vi "ZS_DPLab_Main_ver3.1.vi"() -> ()   [LabVIEW 2011]
panel:
  in  "File type":u16(ring) items=["Txt"=0, "Both"=2]
  out "StartTime(ms)":u32
  in  "Pause":bool
  in  "stop":bool
  in  "Main Sweep":u8(ring) items=["Time", "DC Current", "Delta Current", "Pulse Delta Current", "Sine Current", "Lock-In Vosc"]
  out "Run index":string
  in  "File Index:":u16=1 format="%03d"
  out "TakingData":bool
  in  "Data File Address":path
  in  "Tab Control":T1(tab)
  in  "Steps Config:":T2={"# of points:"=100, "Step Delay (s)"=1.0, "Ini Delay (s)"=3.0, "# of steps:"=1} {"# of steps:" step=1; "# of points:" step=1; "Step Delay (s)" min=0.0 format="%3.2f"; "Ini Delay (s)" min=0.0 format="%3.2f"}
  in  "Tab Control 2":enum32{"ITC 503", "LS 340"}(tab)
  in  "Temperature Control (ITC 503):":T3={"GPIB ADR"=0, "Change Heater?"={"Change Heater?"=FALSE, "Heater"=0}, "Change Temp?"={"Change Temp?"=FALSE, "Set Temp (K)"=0.0}, "Cluster"={"Heat Auto?"=FALSE, "Manual Heat?"=FALSE, "Heater Manual (%)"=0.0}, "Change PID?"={"Change PID?"=FALSE, "Proportional"=0.0, "Integral"=0.0, "Derivative"=0.0}, "Change Para?"=FALSE, "ITC503 Control Sensor"=1} {"ITC503 Control Sensor" items=["T2", "T3"]; "Change PID?"."Derivative" format="%.2f"; "Change PID?"."Integral" format="%.2f"; "Change PID?"."Proportional" format="%.2f"; "Cluster"."Heater Manual (%)" scale=0.0..100.0; "Change Temp?"."Set Temp (K)" format="%.3f"; "Change Heater?"."Heater" items=["Heater 1", "Heater 2", "Heater 3"]; "GPIB ADR" items=["None"=0, "24"=24]}
  in  "Temperature Control (LS 340):":T4={"GPIB ADR"=0, "From (K)"=0.0, "To (K)"=0.0, "Rate (K/min; 0~100)"=1.0, "Delta T (0.08K)"=0.08, "Temp. Header"="Temp_K", "Temp. Display controller"={"Ch B"=TRUE, "Ch C"=TRUE, "Ch D"=FALSE}} {"Delta T (0.08K)" format="%.3f"; "Rate (K/min; 0~100)" format="%.1f"; "To (K)" format="%.2f"; "From (K)" format="%.2f"; "GPIB ADR" items=["None"=0, "30"=30]}
  in  "Measuring Instruments :":T5(array[cluster])
  in  "Keithley 6221 :":T6(array[cluster]) {"Sweep Mode" items=["Linear", "Log", "Exp", "Inverse", "Manual"]; "GPIB ADR" items=["None"=0, "12"=12, "13"=13]; "To I_Sin (A)" format="%#.5p"; "To I_H (A)" format="%#.5p"; "To I_HI (A)" format="%#.5p"; "To I (A)" format="%#.5p"; "Delay (s)" format="%.3p"; "Pulse Width (s)" format="%.3p"; "Delay Time (s)" format="%#.5p"; "DC Offset (A)" format="%#.5p"; "From I_Sin (A)" format="%#.5p"; "Freq (Hz)" format="%#_6p"; "I_L (A)" format="%#.5p"; "From I_H (A)" format="%#.5p"; "I_LO (A)" format="%#.5p"; "From I (A)" format="%#.5p"; "From I_HI (A)" format="%#.5p"}
  in  "Lock-In SR7265 :":T7(array[cluster]) {"Sweep Mode" items=["Linear", "Log", "Exp", "Inverse", "Manual"]; "To" format="%#.5p"; "From" format="%#.5p"; "GPIB ADR" items=["None"=0, "11"=11, "16"=16]}
  in  "Description of this measurement":string
  in  "Varialbe Instruments:":i32(listbox)
  in  "Instruments Config:":string[][](table) caption="Table"
  out "Configuration Profile:":string
  in  "Up Button":bool
  in  "Delete Button":bool
  in  "Down Button":bool
  in  "Add one Run":bool
  in  "Tab Control 3":enum32{"ReadMe", "Control Panel"}(tab)
  in  "Magnet Control (IPS 120-10)":T8={"Action"=1, "Standby (s)"=0.0, "Heater on (s)"=300.0, "Sweep Setup "=[], "GPIB ADR"=0, "Change Para?"=FALSE} {"GPIB ADR" items=["None"=0, "25"=25]; "Sweep Setup"."Hold(min)" min=0.0; "Sweep Setup"."Set Rate(T/min)" min=0.001 max=0.5 step=0.001; "Sweep Setup"."Set Point (T)" min=-9.0 max=9.0 step=0.001; "Action" items=["Hold", "To Set Point", "To Zero", "Clamp"]}
  in  "SettingGo":bool
  in  "Discarded pts":i32
  in  "Analysis":bool=TRUE
  in  "Measure with H/T sweep?":bool=TRUE
  in  "Run Batch Array":T9(array[cluster]) {"Main Sweep" items=["Time", "DC Current", "Delta Current", "Pulse Delta Current", "Sine Current", "Lock-in Vosc"]; "Temperature Control (ITC 503):"."Sensor" items=["T2", "T3"]; "Magnet Control (IPS 120-10)"."Action" items=["Hold", "To Set point", "To Zero", "Clamp"]; "Keithley 6221 :"."Sweep Mode" items=["Linear", "Log", "Exp", "Inverse", "Manual"]}
  in  "Delete Run":bool
  in  "BatchSettingGo":bool
  out "T2":string
  out "T3":string
  out "B":string
  out "T1":string
  in  "DisplayControl":T10 {"Scale" items=["L", "R"]; "Y - axes"."Y 6" items=["", "Time_sec", "T2_K", "T3_K", "I_DeltaHigh_A", "V_Delta_V", "CernoxV_V"]; "Y - axes"."Y 5" items=["", "Time_sec", "T2_K", "T3_K", "I_DeltaHigh_A", "V_Delta_V", "CernoxV_V"]; "Y - axes"."Y 4" items=["", "Time_sec", "T2_K", "T3_K", "I_DeltaHigh_A", "V_Delta_V", "CernoxV_V"]; "Y - axes"."Y 3" items=["", "Time_sec", "T2_K", "T3_K", "I_DeltaHigh_A", "V_Delta_V", "CernoxV_V"]; "Y - axes"."Y 2" items=["", "Time_sec", "T2_K", "T3_K", "I_DeltaHigh_A", "V_Delta_V", "CernoxV_V"]; "Y - axes"."Y 1" items=["", "Time_sec", "T2_K", "T3_K", "I_DeltaHigh_A", "V_Delta_V", "CernoxV_V"]; "X - axis" items=["Time_sec", "T2_K", "T3_K", "I_DeltaHigh_A", "V_Delta_V", "CernoxV_V"]}
  out "XY Graph":cluster{"DataOut":dbl[], "DataOut":dbl[]}[](graph)
  out "DataDisplay":T11
  out "Set T:":string
  out "Set B:":string
  out "Title Name Array":string[](array[string])
  out "Data Table":dbl[][](array[numeric])
  out "XY Graph 2":cluster{"DataOut":dbl[], "DataOut":dbl[]}[](graph)
  in  "AnalysisDisplayControl":T10 {"Scale" items=["L", "R"]; "Y - axes"."Y 6" items=["", "Time_sec", "T2_K", "Std_T2_K", "T3_K", "Std_T3_K", "I_DeltaHigh_A", "Std_I_DeltaHigh_A", "V_Delta_V", "Std_V_Delta_V", "CernoxV_V", "Std_CernoxV_V", "CernoxR_Ohms", "Std_CernoxR_Ohms", "CernoxT_K", "Std_CernoxT_K"]; "Y - axes"."Y 5" items=["", "Time_sec", "T2_K", "Std_T2_K", "T3_K", "Std_T3_K", "I_DeltaHigh_A", "Std_I_DeltaHigh_A", "V_Delta_V", "Std_V_Delta_V", "CernoxV_V", "Std_CernoxV_V", "CernoxR_Ohms", "Std_CernoxR_Ohms", "CernoxT_K", "Std_CernoxT_K"]; "Y - axes"."Y 4" items=["", "Time_sec", "T2_K", "Std_T2_K", "T3_K", "Std_T3_K", "I_DeltaHigh_A", "Std_I_DeltaHigh_A", "V_Delta_V", "Std_V_Delta_V", "CernoxV_V", "Std_CernoxV_V", "CernoxR_Ohms", "Std_CernoxR_Ohms", "CernoxT_K", "Std_CernoxT_K"]; "Y - axes"."Y 3" items=["", "Time_sec", "T2_K", "Std_T2_K", "T3_K", "Std_T3_K", "I_DeltaHigh_A", "Std_I_DeltaHigh_A", "V_Delta_V", "Std_V_Delta_V", "CernoxV_V", "Std_CernoxV_V", "CernoxR_Ohms", "Std_CernoxR_Ohms", "CernoxT_K", "Std_CernoxT_K"]; "Y - axes"."Y 2" items=["", "Time_sec", "T2_K", "Std_T2_K", "T3_K", "Std_T3_K", "I_DeltaHigh_A", "Std_I_DeltaHigh_A", "V_Delta_V", "Std_V_Delta_V", "CernoxV_V", "Std_CernoxV_V", "CernoxR_Ohms", "Std_CernoxR_Ohms", "CernoxT_K", "Std_CernoxT_K"]; "Y - axes"."Y 1" items=["", "Time_sec", "T2_K", "Std_T2_K", "T3_K", "Std_T3_K", "I_DeltaHigh_A", "Std_I_DeltaHigh_A", "V_Delta_V", "Std_V_Delta_V", "CernoxV_V", "Std_CernoxV_V", "CernoxR_Ohms", "Std_CernoxR_Ohms", "CernoxT_K", "Std_CernoxT_K"]; "X - axis" items=["Time_sec", "T2_K", "Std_T2_K", "T3_K", "Std_T3_K", "I_DeltaHigh_A", "Std_I_DeltaHigh_A", "V_Delta_V", "Std_V_Delta_V", "CernoxV_V", "Std_CernoxV_V", "CernoxR_Ohms", "Std_CernoxR_Ohms", "CernoxT_K", "Std_CernoxT_K"]}
  in  "Cernox T Fitting Control":T12={"Cernox V title"="CernoxV_V", "Cernox I title"="CernoxI_V", "Cernox V Lockin Sen (V)"=0.001, "Cernox I Lockin Sensitivity (V)"=0.02, "Cernox I Current Amp Sen (A/V)"=1e-05, "Cernox Fit"=TRUE}
  in  "CernoxI measured with a lock-in?":bool
  in  "Cernox_I":dbl=4.965
  # "If set rate = 0,                           Ramping is off."
  # "If set temp. = 0,    \nThe Temp. is not controlled."
  # "Before you start:\n1. Make sure you finished the training and authorized to use this magnet.\n2. Check Helium level of the cryostat before you proceed. Generally you should sweep field back to zero if the level is below 16%.\n3. This module is designed for normal sweep mode, so make sure the \"SWITCH HEATER\" is \"SELECT\" and \"CONFIRM\". If you need the persistent mode, please control IPS manualy.\n4. This module is adopted from Xiaoyan_IPS_120_10 ver2.0-2.vi. Please make sure you are absolutely familiar with all the settings before you start to set up the batch files.\n5. Recommended B sweep rate is ~ 0.1 T/min."
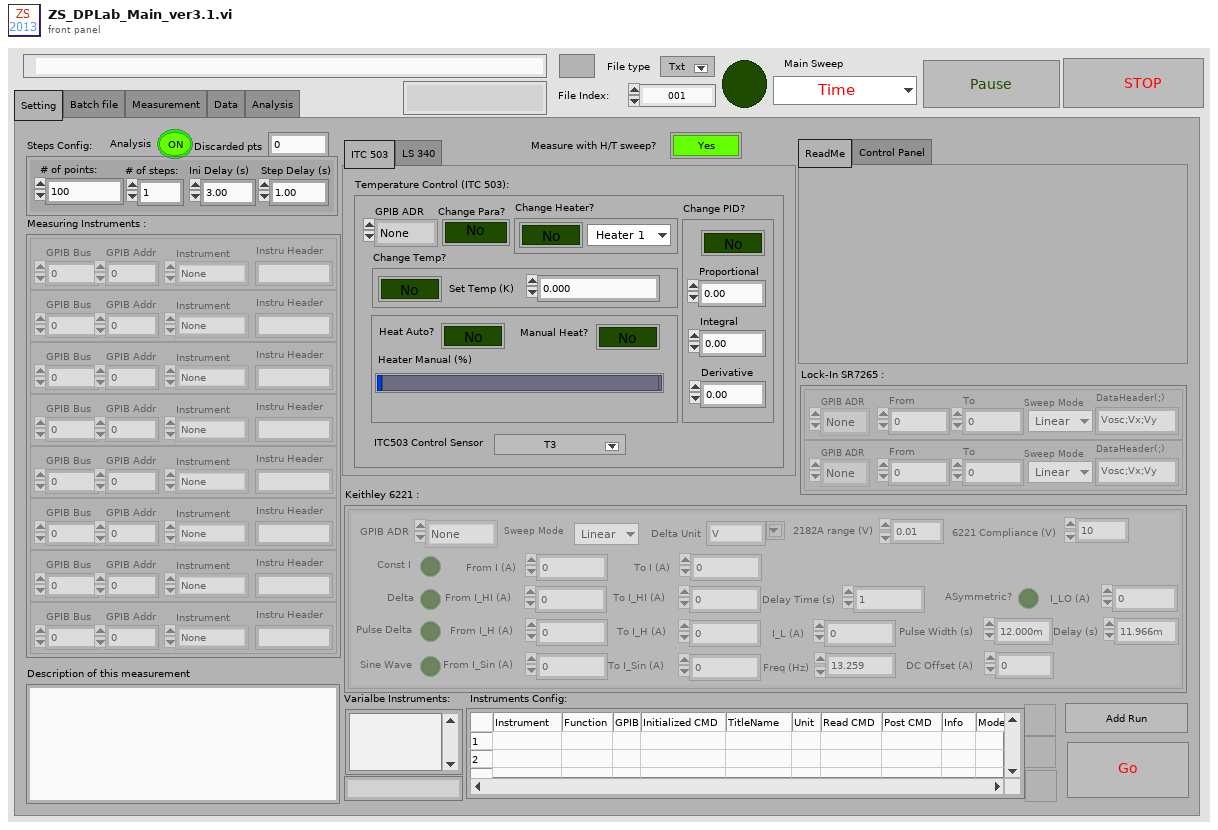
[diagram p1: front panel]
types:
  T1 = enum32{"Setting", "Batch file", "Measurement", "Data", "Analysis"}
  T2 = cluster{"# of points:":u32, "Step Delay (s)":dbl, "Ini Delay (s)":dbl, "# of steps:":u32}
  T3 = cluster{"GPIB ADR":u16, "Change Heater?":cluster{"Change Heater?":bool, "Heater":u8}, "Change Temp?":cluster{"Change Temp?":bool, "Set Temp (K)":dbl}, "Cluster":cluster{"Heat Auto?":bool, "Manual Heat?":bool, "Heater Manual (%)":dbl}, "Change PID?":cluster{"Change PID?":bool, "Proportional":dbl, "Integral":dbl, "Derivative":dbl}, "Change Para?":bool, "ITC503 Control Sensor":u16}
  T4 = cluster{"GPIB ADR":u16, "From (K)":dbl, "To (K)":dbl, "Rate (K/min; 0~100)":dbl, "Delta T (0.08K)":dbl, "Temp. Header":string, "Temp. Display controller":cluster{"Ch B":bool, "Ch C":bool, "Ch D":bool}}
  T5 = cluster{"GPIB Bus":dbl, "GPIB Addr":dbl, "Instrument":enum16{"None", "HP34401DMM", "Lockin 7265", "HP3456/7A", "HP3478A", "HP3325FG", "Keithley2182A"}, "Instru Header":string}[]
  T6 = cluster{"Delta ":bool, "Const I ":bool, "Pulse Delta ":bool, "Sine Wave ":bool, "From I_HI (A)":dbl, "From I (A)":dbl, "I_LO (A)":dbl, "From I_H (A)":dbl, "I_L (A)":dbl, "Freq (Hz)":dbl, "From I_Sin (A)":dbl, "DC Offset (A)":dbl, "Delay Time (s)":dbl, "Pulse Width (s)":dbl, "Delay (s)":dbl, "To I (A)":dbl, "ASymmetric?":bool, "To I_HI (A)":dbl, "To I_H (A)":dbl, "To I_Sin (A)":dbl, "GPIB ADR":u16, "Sweep Mode":u8, "Delta Unit":string, "2182A range (V)":dbl, "6221 Compliance (V)":dbl}[]
  T7 = cluster{"GPIB ADR":u16, "From":dbl, "To":dbl, "DataHeader(;)":string, "Sweep Mode":u8}[]
  T8 = cluster{"Action":u16, "Standby (s)":dbl, "Heater on (s)":dbl, "Sweep Setup ":cluster{"Set Point (T)":dbl, "Set Rate(T/min)":dbl, "Hold(min)":dbl}[], "GPIB ADR":u16, "Change Para?":bool}
  T9 = cluster{"Main Sweep":u8, "Steps Config:":cluster{"total points:":u32, "Step Delay (s)":dbl, "Ini Delay (s)":dbl, "# of steps:":u32}, "Temperature Control (ITC 503):":cluster{"GPIB ADR":u16, "Change Heater?":cluster{"Heater?":bool, "Heater":u8}, "Change Temp?":cluster{"Change T?":bool, "Set T (K)":dbl}, "Cluster":cluster{"Heat Auto?":bool, "Manual Heat?":bool, "Heater (%)":dbl}, "Change PID?":cluster{"Change PID?":bool, "P":dbl, "I":dbl, "D":dbl}, "Change Para?":bool, "Sensor":u16}, "Temperature Control (LS 340):":cluster{"GPIB ADR":u16, "From (K)":dbl, "To (K)":dbl, "Rate (K/min)":dbl, "Delta T (0.08K)":dbl, "Temp. Header":string, "T Display Control":cluster{"Ch B":bool, "Ch C":bool, "Ch D":bool}}, "Magnet Control (IPS 120-10)":cluster{"Action":u16, "Standby (s)":dbl, "Heater on (s)":dbl, "Sweep Setup ":cluster{"Set Point (T)":dbl, "Set Rate(T/min)":dbl, "Hold(min)":dbl}[], "GPIB ADR":u16, "Change Para?":bool}, "Keithley 6221 :":cluster{"Delta mode":bool, "Const I":bool, "Pulse Delta mode":bool, "Sine Wave Mode":bool, "From I_HI (A)":dbl, "From I (A)":dbl, "I_LO (A)":dbl, "From I_H (A)":dbl, "I_L (A)":dbl, "Freq (Hz)":dbl, "From I_Sin (A)":dbl, "DC Offset (A)":dbl, "Delay Time (s)":dbl, "Pulse Width (s)":dbl, "Delay (s)":dbl, "To I (A)":dbl, "ASymmetric?":bool, "To I_HI (A)":dbl, "To I_H (A)":dbl, "To I_Sin (A)":dbl, "GPIB ADR":u16, "Sweep Mode":u8, "Delta Unit":string, "2182A range (V)":dbl, "6221 Compliance (V)":dbl}[], "Measuring Instruments : ":cluster{"GPIB Bus":dbl, "GPIB Addr":dbl, "Instrument":enum16{"None", "HP34401DMM", "Lockin 7265", "HP3456/7A", "HP3478A", "HP3325FG", "Keithley2182A"}, "Instru Header":string}[], "Lock-In SR7265 :":cluster{"GPIB ADR":u16, "From":dbl, "To":dbl, "Header(;)":string, "Sweep Mode":u8}[], "Deascription of \nthis measurement":string, "Instruments Config:":string[][]}[]
  T10 = cluster{"X - axis":u8, "Y - axes":cluster{"Y 1":u8, "Y 2":u8, "Y 3":u8, "Y 4":u8, "Y 5":u8, "Y 6":u8}, "Scale":u16[]}
  T11 = cluster{"X":dbl, "Y 1":dbl, "Y 2":dbl, "Y 3":dbl, "Y 4":dbl, "Y 5":dbl, "Y 6":dbl}
  T12 = cluster{"Cernox V title":string, "Cernox I title":string, "Cernox V Lockin Sen (V)":dbl, "Cernox I Lockin Sensitivity (V)":dbl, "Cernox I Current Amp Sen (A/V)":dbl, "Cernox Fit":bool}
  T13 = cluster{"Main Sweep":u8, "Steps Config:":cluster{"total points:":u32, "Step Delay (s)":dbl, "Ini Delay (s)":dbl, "# of steps:":u32}, "Temperature Control (ITC 503):":cluster{"GPIB ADR":u16, "Change Heater?":cluster{"Heater?":bool, "Heater":u8}, "Change Temp?":cluster{"Change T?":bool, "Set T (K)":dbl}, "Cluster":cluster{"Heat Auto?":bool, "Manual Heat?":bool, "Heater (%)":dbl}, "Change PID?":cluster{"Change PID?":bool, "P":dbl, "I":dbl, "D":dbl}, "Change Para?":bool, "Sensor":u16}, "Temperature Control (LS 340):":cluster{"GPIB ADR":u16, "From (K)":dbl, "To (K)":dbl, "Rate (K/min)":dbl, "Delta T (0.08K)":dbl, "Temp. Header":string, "T Display Control":cluster{"Ch B":bool, "Ch C":bool, "Ch D":bool}}, "Magnet Control (IPS 120-10)":cluster{"Action":u16, "Standby (s)":dbl, "Heater on (s)":dbl, "Sweep Setup ":cluster{"Set Point (T)":dbl, "Set Rate(T/min)":dbl, "Hold(min)":dbl}[], "GPIB ADR":u16, "Change Para?":bool}, "Keithley 6221 :":cluster{"Delta mode":bool, "Const I":bool, "Pulse Delta mode":bool, "Sine Wave Mode":bool, "From I_HI (A)":dbl, "From I (A)":dbl, "I_LO (A)":dbl, "From I_H (A)":dbl, "I_L (A)":dbl, "Freq (Hz)":dbl, "From I_Sin (A)":dbl, "DC Offset (A)":dbl, "Delay Time (s)":dbl, "Pulse Width (s)":dbl, "Delay (s)":dbl, "To I (A)":dbl, "ASymmetric?":bool, "To I_HI (A)":dbl, "To I_H (A)":dbl, "To I_Sin (A)":dbl, "GPIB ADR":u16, "Sweep Mode":u8, "Delta Unit":string, "2182A range (V)":dbl, "6221 Compliance (V)":dbl}[], "Measuring Instruments : ":cluster{"GPIB Bus":dbl, "GPIB Addr":dbl, "Instrument":enum16{"None", "HP34401DMM", "Lockin 7265", "HP3456/7A", "HP3478A", "HP3325FG", "Keithley2182A"}, "Instru Header":string}[], "Lock-In SR7265 :":cluster{"GPIB ADR":u16, "From":dbl, "To":dbl, "Header(;)":string, "Sweep Mode":u8}[], "Deascription of \nthis measurement":string, "Instruments Config:":string[][]}
  T14 = enum32{"Setting", "Batch file", "Measurement", "Data"}
  T15 = cluster{"Main Sweep":u8, "Steps Config:":cluster{"# of points:":u32, "Step Delay (s)":dbl, "Ini Delay (s)":dbl, "# of steps:":u32}, "Temperature Control (ITC 503):":cluster{"GPIB ADR":u16, "Change Heater?":cluster{"Change Heater?":bool, "Heater":u8}, "Change Temp?":cluster{"Change Temp?":bool, "Set Temp (K)":dbl}, "Cluster":cluster{"Heat Auto?":bool, "Manual Heat?":bool, "Heater Manual (%)":dbl}, "Change PID?":cluster{"Change PID?":bool, "Proportional":dbl, "Integral":dbl, "Derivative":dbl}, "Change Para?":bool, "ITC503 Control Sensor":u16}, "Temperature Control (LS 340):":cluster{"GPIB ADR":u16, "From (K)":dbl, "To (K)":dbl, "Rate (K/min; 0~100)":dbl, "Delta T (0.08K)":dbl, "Temp. Header":string, "Temp. Display controller":cluster{"Ch B":bool, "Ch C":bool, "Ch D":bool}}, "Magnet Control (IPS 120-10)":cluster{"Action":u16, "Standby (s)":dbl, "Heater on (s)":dbl, "Sweep Setup ":cluster{"Set Point (T)":dbl, "Set Rate(T/min)":dbl, "Hold(min)":dbl}[], "GPIB ADR":u16, "Change Para?":bool}, "Keithley 6221 :":cluster{"Delta ":bool, "Const I ":bool, "Pulse Delta ":bool, "Sine Wave ":bool, "From I_HI (A)":dbl, "From I (A)":dbl, "I_LO (A)":dbl, "From I_H (A)":dbl, "I_L (A)":dbl, "Freq (Hz)":dbl, "From I_Sin (A)":dbl, "DC Offset (A)":dbl, "Delay Time (s)":dbl, "Pulse Width (s)":dbl, "Delay (s)":dbl, "To I (A)":dbl, "ASymmetric?":bool, "To I_HI (A)":dbl, "To I_H (A)":dbl, "To I_Sin (A)":dbl, "GPIB ADR":u16, "Sweep Mode":u8, "Delta Unit":string, "2182A range (V)":dbl, "6221 Compliance (V)":dbl}[], "Measuring Instruments : ":cluster{"GPIB Bus":dbl, "GPIB Addr":dbl, "Instrument":enum16{"None", "HP34401DMM", "Lockin 7265", "HP3456/7A", "HP3478A", "HP3325FG", "Keithley2182A"}, "Instru Header":string}[], "Lock-In SR7265 :":cluster{"GPIB ADR":u16, "From":dbl, "To":dbl, "DataHeader(;)":string, "Sweep Mode":u8}[], "Description of this measurement":string, "Instruments Config:":string[][]}
  T16 = typedef "LVRowAndColumnTypeDef.ctl" = cluster{"Row":i32, "Column":i32}
  T17 = cluster{"Delta mode":bool, "Const I":bool, "Pulse Delta mode":bool, "Sine Wave Mode":bool, "From I_HI (A)":dbl, "From I (A)":dbl, "I_LO (A)":dbl, "From I_H (A)":dbl, "I_L (A)":dbl, "Freq (Hz)":dbl, "From I_Sin (A)":dbl, "DC Offset (A)":dbl, "Delay Time (s)":dbl, "Pulse Width (s)":dbl, "Delay (s)":dbl, "To I (A)":dbl, "ASymmetric?":bool, "To I_HI (A)":dbl, "To I_H (A)":dbl, "To I_Sin (A)":dbl, "GPIB ADR":u16, "Sweep Mode":u8, "Delta Unit":string, "2182A range (V)":dbl, "6221 Compliance (V)":dbl}[]
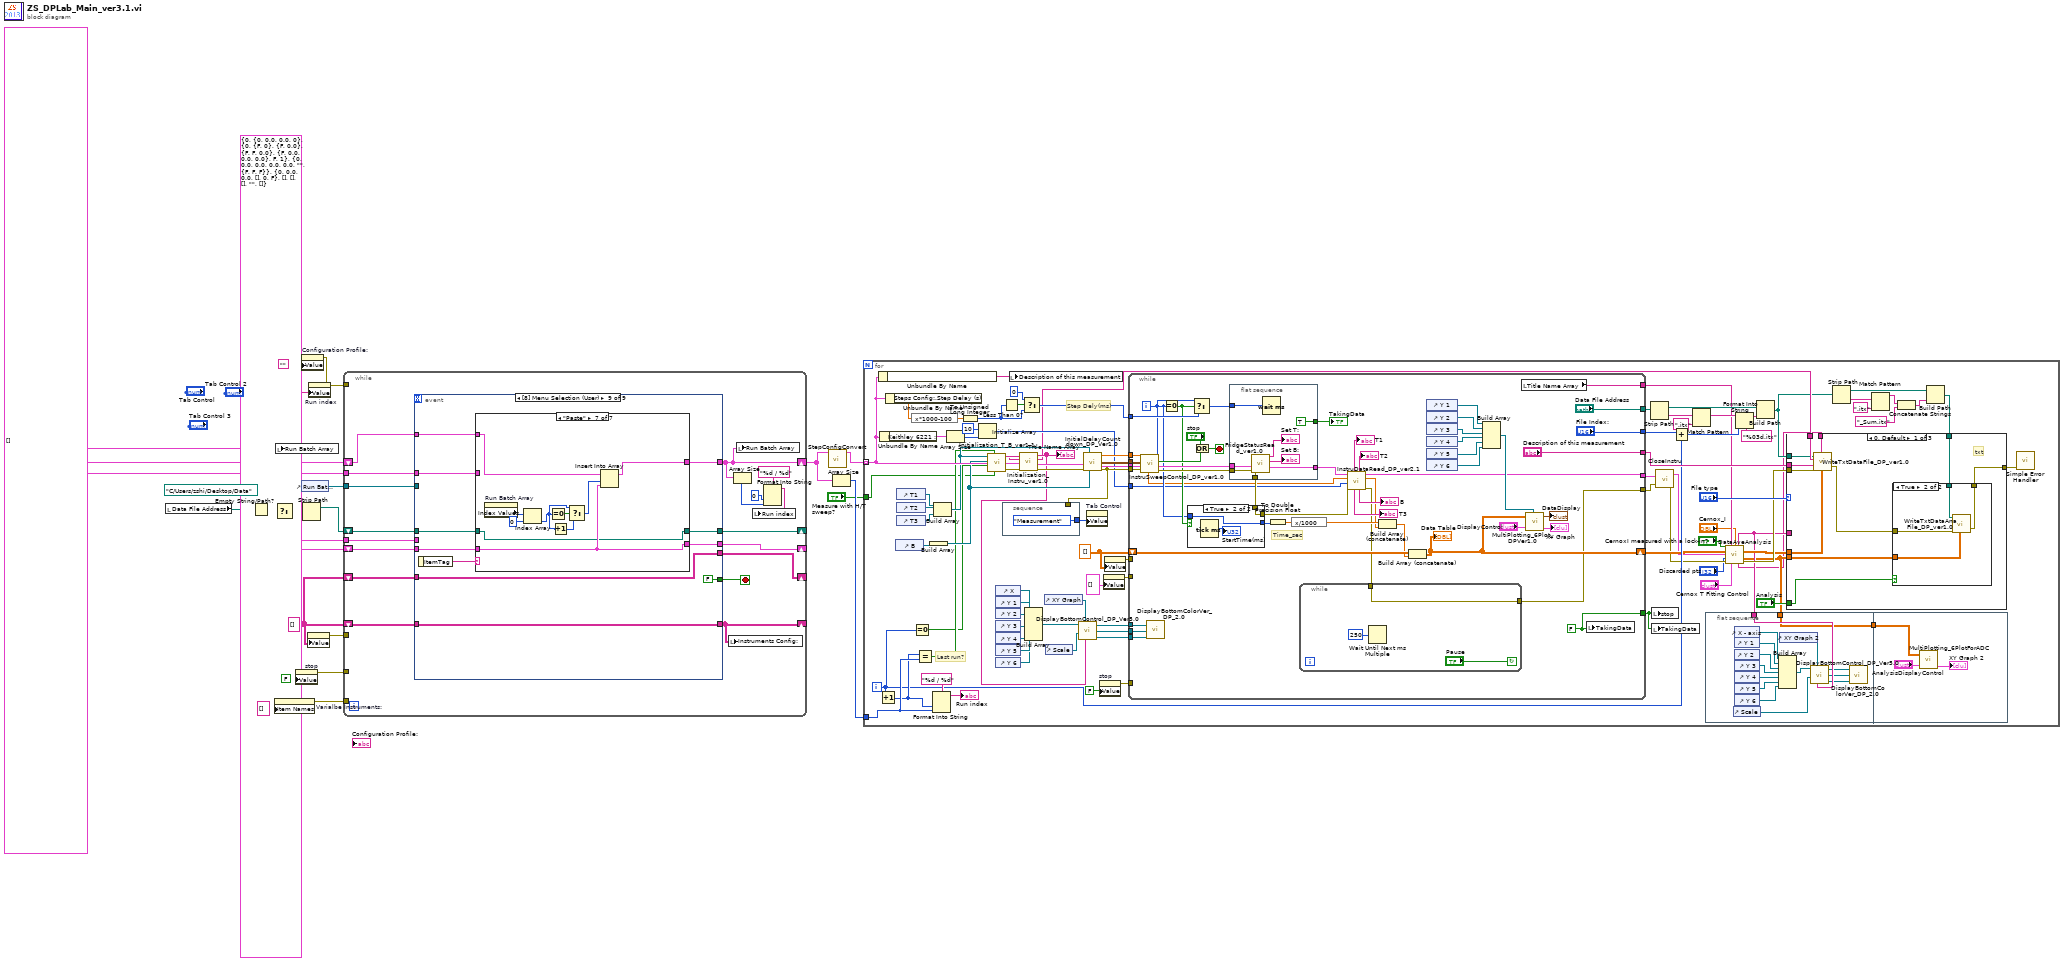
[diagram p0: block diagram]
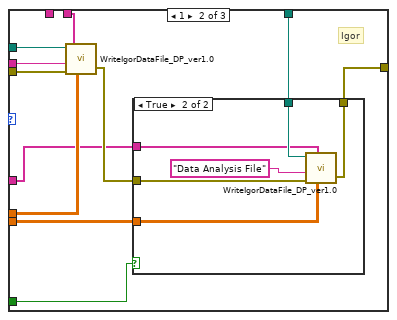
[diagram p3: hidden frame]
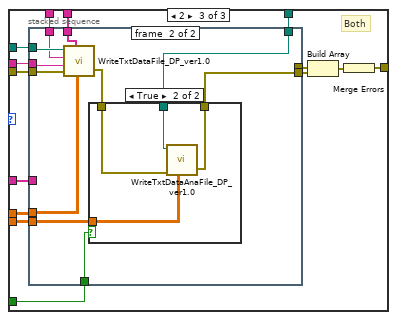
[diagram p5: hidden frame]
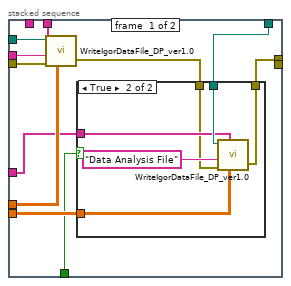
[diagram p6: hidden frame]
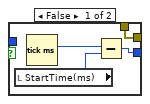
[diagram p9: hidden frame]
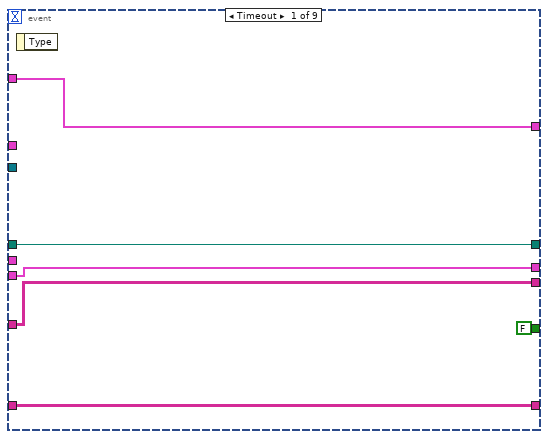
[diagram p10: hidden frame]
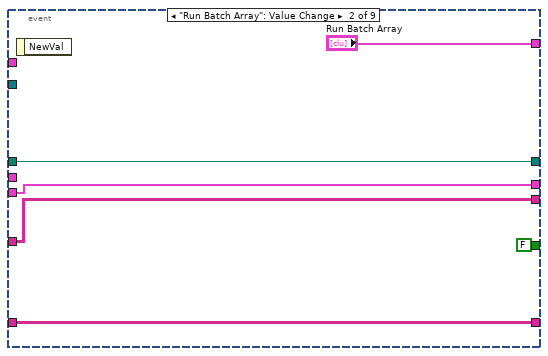
[diagram p11: hidden frame]
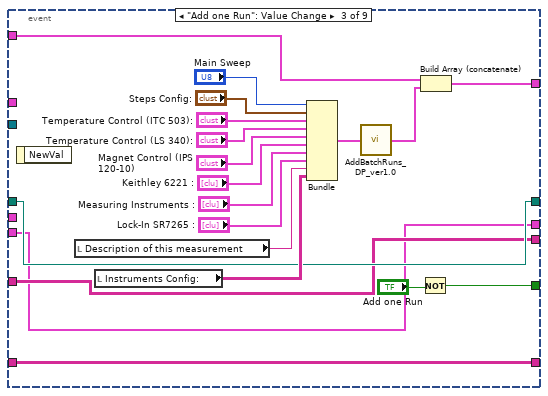
[diagram p12: hidden frame]
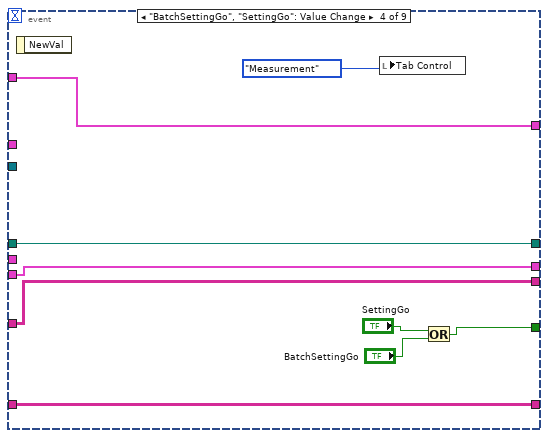
[diagram p13: hidden frame]
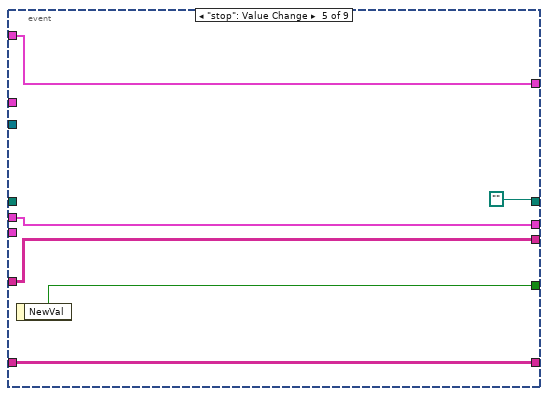
[diagram p14: hidden frame]
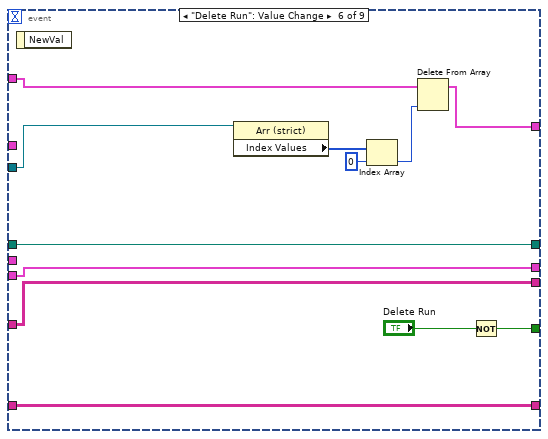
[diagram p15: hidden frame]
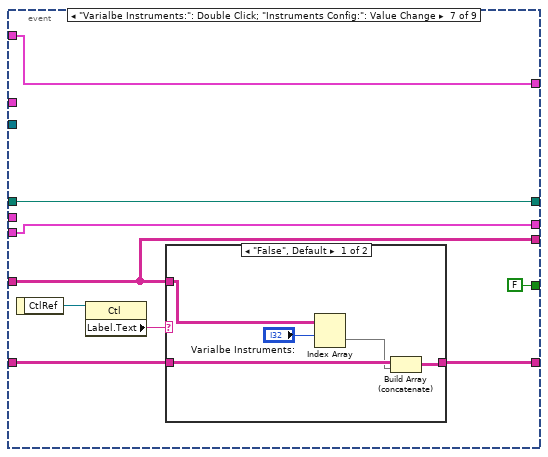
[diagram p16: hidden frame]
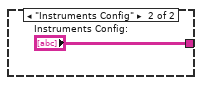
[diagram p17: hidden frame]
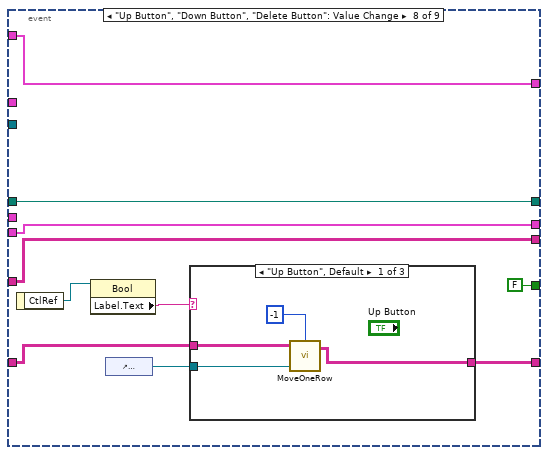
[diagram p18: hidden frame]
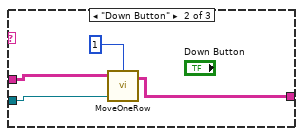
[diagram p19: hidden frame]
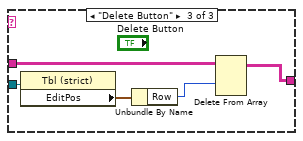
[diagram p20: hidden frame]
diagram:
  w2 = T13 {"Main Sweep"=0, "Steps Config:"={"total points:"=0, "Step Delay (s)"=0.0, "Ini Delay (s)"=0.0, "# of steps:"=0}, "Temperature Control (ITC 503):"={"GPIB ADR"=0, "Change Heater?"={"Heater?"=FALSE, "Heater"=0}, "Change Temp?"={"Change T?"=FALSE, "Set T (K)"=0.0}, "Cluster"={"Heat Auto?"=FALSE, "Manual Heat?"=FALSE, "Heater (%)"=0.0}, "Change PID?"={"Change PID?"=FALSE, "P"=0.0, "I"=0.0, "D"=0.0}, "Change Para?"=FALSE, "Sensor"=1}, "Temperature Control (LS 340):"={"GPIB ADR"=0, "From (K)"=0.0, "To (K)"=0.0, "Rate (K/min)"=0.0, "Delta T (0.08K)"=0.0, "Temp. Header"="", "T Display Control"={"Ch B"=FALSE, "Ch C"=FALSE, "Ch D"=FALSE}}, "Magnet Control (IPS 120-10)"={"Action"=0, "Standby (s)"=0.0, "Heater on (s)"=0.0, "Sweep Setup "=[], "GPIB ADR"=0, "Change Para?"=FALSE}, "Keithley 6221 :"=[], "Measuring Instruments : "=[], "Lock-In SR7265 :"=[], "Deascription of \nthis measurement"="", "Instruments Config:"=[]} ("output cluster")
  w3 = T9 [] ("Run Batch Array 2")
  w13 = ""
  w19 = string[][] [] ("Instruments Config:")
  n1 = local read "Data File Address"() -> (w16:path)
  n2 = Empty String/Path?(string/path=w16) -> (empty?=w18:bool)
  n3 = property on="Varialbe Instruments:" class="LstBox (strict)"("Item Names"=string[] []) -> (error out=w10:errorcluster)  [unwired: 2 in, 1 out]
  n4 = local write "Run Batch Array"(w3) -> ()
  n5 = Select(t=path "C:/Users/zshi/Desktop/Data" ("Data File Address"), s=w18, f=w16) -> (s? t:f=w15:path)
  n6 = property on="stop" class="Bool (strict)"("Value"=FALSE ("stop")) -> (error out=w6:errorcluster)  [unwired: 2 in, 1 out]
  n7 = control-ref of="Run Batch Array"() -> (w21:refnum<vi>)
  n8 = property on="Configuration Profile:" class="Str"("Value"=w13) -> (error out=w12:errorcluster)  [unwired: 2 in, 1 out]
  n9 = Strip Path(path=w15) -> (stripped path=w14:path)  [unwired: 1 out]
  n10 = property on="Instruments Config:" class="Tbl (strict)"("Value"=w19) -> (error out=w20:errorcluster)  [unwired: 2 in, 1 out]
  n11 = property on="Run index" class="Str"(error in=w12, "Value"=w13) -> (error out=w11:errorcluster)  [unwired: 1 in, 1 out]
  n12 = while {
    shift-right: [w26] -> w5
    shift-left: w3 -> [w38]
    tunnel: w21 -> [w37]
    shift-right: [w36] -> _
    shift-left: w19 -> [w34]
    tunnel: w20 -> [_]
    shift-right: [w33] -> _
    shift-left: w19 -> [w35]
    shift-right: [w27] -> _
    shift-left: w14 -> [w28]
    tunnel: w11 -> [_]
    tunnel: w10 -> [_]
    tunnel: w6 -> [_]
    tunnel: w3 -> [w25]
    shift-right: [w24] -> _
    shift-left: w2 -> [w23]
    tunnel: w2 -> [w22]
    stop <- w39 stop-if-true
    n13 = event shown="[8] Menu Selection (User)" {
      selector: _ -> [_ _ _ _ _ _ _ _ _]
      dyn-events: _ -> [_ _ _ _ _ _ _ _ _]
      timeout: _ -> [_ _ _ _ _ _ _ _ _]
      tunnel: [FALSE FALSE w61 w77 w86 w97 FALSE ("NewVal") FALSE ("NewVal") FALSE ("NewVal")] -> w39
      tunnel: w38 -> [w44 _ w60 w80 w85 w92 w101 w116 w144]
      tunnel: [w44 "Run Batch Array" w59 w80 w85 w91 w101 w116 w145] -> w26
      tunnel: w37 -> [_ _ _ _ _ w96 _ _ _]
      tunnel: [w41 w47 w56 w74 w83 w88 w105 w117 w138] -> w36
      tunnel: w35 -> [w42 w48 w57 w75 w84 w89 w103 w119 w139]
      tunnel: w34 -> [w41 w47 w56 w74 w83 w88 w104 w118 w138]
      tunnel: [w42 w48 w57 w75 w84 w89 w103 w119 w139] -> w33
      tunnel: w28 -> [w43 w49 w58 w76 _ w90 w100 w115 w143]
      tunnel: [w43 w49 w58 w76 path "" w90 w100 w115 w142] -> w27
      tunnel: w25 -> [_ _ _ _ _ _ _ _ w146]
      tunnel: [w40 w46 w52 w72 w81 w87 w99 w114 w141] -> w24
      tunnel: w23 -> [w40 w46 w52 w72 _ w87 w99 w114 w140]
      tunnel: w22 -> [_ _ _ _ w81 _ _ _ _]
      event Timeout {
        n14 = event-data() -> ()  [unwired: 1 in, 1 out]
      }
      event "Run Batch Array": Value Change {
        n15 = event-data() -> ()  [unwired: 1 in, 1 out]
      }
      event "Add one Run": Value Change {
        n16 = event-data() -> ()  [unwired: 1 in, 1 out]
        n17 = local read "Description of this measurement"() -> (w64:string)
        n18 = local read "Instruments Config:"() -> (w63:string[][])
        n19 = Bundle("Main Sweep"="Main Sweep", "Steps Config:"="Steps Config:", "Temperature Control (ITC 503):"="Temperature Control (ITC 503):", "Temperature Control (LS 340):"="Temperature Control (LS 340):", "Magnet Control (IPS 120-10)"="Magnet Control (IPS 120-10)", "Keithley 6221 :"="Keithley 6221 :", "Measuring Instruments :"="Measuring Instruments :", "Lock-In SR7265 :"="Lock-In SR7265 :", "Description of this measurement"=w64, "Instruments Config:"=w63) -> (w55:T15)  [unwired: 1 in]
        n20 = call "AddBatchRuns_DP_ver1.0.vi"("output cluster"=w55) -> ("output cluster 2"=w54:T13)
        n21 = Not(x="Add one Run") -> (.not. x?=w61:bool)
        n22 = Build Array (concatenate)(w60, w54) -> (w59:T9)
      }
      event "BatchSettingGo", "SettingGo": Value Change {
        n23 = event-data() -> ()  [unwired: 1 in, 1 out]
        n24 = local write "Tab Control"(T14."Measurement" ("Tab Control")) -> ()
        n25 = Or(x="SettingGo", y="BatchSettingGo") -> (x .or. y?=w77:bool)
      }
      event "stop": Value Change {
        n26 = event-data() -> ("NewVal"=w86:bool)  [unwired: 1 in]
      }
      event "Delete Run": Value Change {
        n27 = event-data() -> ()  [unwired: 1 in, 1 out]
        n28 = property class="Arr (strict)"(reference=w96) -> ("Index Values"=w95:u32[])  [unwired: 1 in, 2 out]
        n29 = Index Array(array=w95, index=0) -> (element=w93:u32)
        n30 = Delete From Array(array=w92, index=w93) -> (array with subset deleted=w91:T9)  [unwired: 1 in, 1 out]
        n31 = Not(x="Delete Run") -> (.not. x?=w97:bool)
      }
      event "Varialbe Instruments:": Double Click; "Instruments Config:": Value Change {
        n32 = event-data() -> ("CtlRef"=w107:refnum<vi>)  [unwired: 1 in]
        n33 = property class="Ctl"(reference=w107) -> ("Label.Text"=w106:string)  [unwired: 1 in, 2 out]
        n34 = case shown="\"False\", Default" w106 {
          tunnel: [w108 "Instruments Config:"] -> w105
          tunnel: w103 -> [w112 _]
          tunnel: w104 -> [w110 _]
          frame "False", Default {
            n35 = Index Array(array=w112, index (row)="Varialbe Instruments:") -> (element=w109:string[])  [unwired: 1 in]
            n36 = Build Array (concatenate)(w110, w109) -> (w108:string[][])
          }
          frame "Instruments Config" {
          }
        }
      }
      event "Up Button", "Down Button", "Delete Button": Value Change {
        n37 = event-data() -> ("CtlRef"=w123:refnum<vi>)  [unwired: 1 in]
        n38 = property class="Bool"(reference=w123) -> ("Label.Text"=w122:string)  [unwired: 1 in, 2 out]
        n39 = control-ref of="Instruments Config:"() -> (w121:refnum<vi>)
        n40 = case shown="\"Up Button\", Default" w122 {
          tunnel: w121 -> [w127 w131 w134]
          tunnel: w118 -> [w125 w130 w135]
          tunnel: [w124 w128 w136] -> w117
          frame "Up Button", Default {
            n41 = call "MoveOneRow.vi"("#ofMoveRows"=-1, "Table In Ref"=w127, "Table In"=w125) -> ("Table Out"=w124:string[][])  [unwired: 2 in]
          }
          frame "Down Button" {
            n42 = call "MoveOneRow.vi"("#ofMoveRows"=1, "Table In Ref"=w131, "Table In"=w130) -> ("Table Out"=w128:string[][])  [unwired: 2 in]
          }
          frame "Delete Button" {
            n43 = property class="Tbl (strict)"(reference=w134) -> ("EditPos"=w133:T16)  [unwired: 1 in, 2 out]
            n44 = Unbundle By Name(w133) -> ("Row"=w132:i32)
            n45 = Delete From Array(array=w135, index (row)=w132) -> (array with subset deleted=w136:string[][])  [unwired: 2 in, 1 out]
          }
        }
      }
      event Menu Selection (User) {
        n46 = event-data() -> ("ItemTag"=w147:string)  [unwired: 1 in]
        n47 = case shown="\"Paste\"" w147 {
          tunnel: w146 -> [w151 _ _ _ _ _ _]
          tunnel: [w151 w153 w159 w163 w169 w176 w182] -> w145
          tunnel: w144 -> [_ _ w159 w163 w170 w176 w183]
          tunnel: w143 -> [w150 w157 w161 w166 w167 w174 w180]
          tunnel: [w149 w154 w160 w164 w167 w174 w180] -> w142
          tunnel: [w148 w152 w158 w162 w168 w175 w181] -> w141
          tunnel: w140 -> [w148 w152 w158 w162 _ _ w181]
          frame "New", Default {
            n48 = Strip Path(path=w150) -> (stripped path=w149:path)  [unwired: 1 out]
          }
          frame "Load" {
            n49 = Strip Path(path=w157) -> (stripped path=w155:path)  [unwired: 1 out]
            n50 = call "BatchFileReadOut_DP.vi"("start path"=w155) -> ("Run Batch Array"=w153:T9, "File Path"=w154:path)  [unwired: 6 in, 1 out]
            n51 = local write "Tab Control"(T1."Batch file" ("Tab Control")) -> ()
          }
          frame "Save" {
            n52 = call "BatchFileWriteIn_DP.vi"("Run Batch Array"=w159, "file path"=w161) -> ("path"=w160:path)  [unwired: 4 in, 2 out]
          }
          frame "Save As" {
            n53 = Strip Path(path=w166) -> (stripped path=w165:path)  [unwired: 1 out]
            n54 = call "BatchFileWriteIn_DP.vi"("start path"=w165, "Run Batch Array"=w163) -> ("path"=w164:path)  [unwired: 4 in, 2 out]
          }
          frame "Cut" {
            n55 = property on="Run Batch Array" class="Arr (strict)"() -> ("Index Values"=w171:u32[])  [unwired: 2 in, 2 out]
            n56 = Index Array(array=w171, index=0) -> (element=w172:u32)
            n57 = Delete From Array(array=w170, index=w172) -> (deleted portion=w168:T13, array with subset deleted=w169:T9)  [unwired: 1 in]
          }
          frame "Copy" {
            n58 = property on="Run Batch Array" class="Arr (strict)"() -> ("Index Values"=w178:u32[])  [unwired: 2 in, 2 out]
            n59 = Index Array(array=w178, index=0) -> (element=w177:u32)
            n60 = Index Array(array=w176, index=w177) -> (element=w175:T13)
          }
          frame "Paste" {
            n61 = property on="Run Batch Array" class="Arr (strict)"() -> ("Index Values"=w188:u32[])  [unwired: 2 in, 2 out]
            n62 = Index Array(array=w188, index=0) -> (element=w185:u32)
            n63 = Equal To 0?(x=w185) -> (x = 0?=w187:bool)
            n64 = Increment(x=w185) -> (x+1=w186:u32)
            n65 = Select(t=w185, s=w187, f=w186) -> (s? t:f=w184:u32)
            n66 = Insert Into Array(array=w183, index=w184, new element=w181) -> (w182:T9)
          }
        }
      }
    }
    n67 = local write "Instruments Config:"(w36) -> ()
    n68 = Array Size(array=w26) -> (size(s)=w31:i32)
    n69 = local write "Run Batch Array"(w26) -> ()
    n70 = Format Into String(format string="%d / %d", 0 ("input 1"), w31) -> (resulting string=w29:string)  [unwired: 2 in, 1 out]
    n71 = local write "Run index"(w29) -> ()
  }
  n72 = call "StepConfigConvert.vi"("Run Batch Array 4"=w5) -> ("Run Batch Array 3"=w4:T9)  [unwired: 10 in]
  n73 = Array Size(array=w5) -> (size(s)=w8:i32)
  n74 = for {
    tunnel: w4 -> [w268] mode=indexing
    tunnel: w8 -> [w221]
    tunnel: "Measure with H/T sweep?" -> [w190]
    i -> [w218]
    w264 = dbl[][] []
    # "Last run?"
    # "Step Dely(ms)"
    n75 = Unbundle By Name(w268) -> ("Deascription of \nthis measurement"=w269:string)
    n76 = Increment(x=w218) -> (x+1=w220:i32)
    n77 = Unbundle By Name(w268) -> ("Keithley 6221 :"=w267:T17)
    n78 = Unbundle By Name(w268) -> ("Steps Config:.Step Delay (s)"=w271:dbl)
    n79 = control-ref of="B"() -> (w242:refnum<vi>)
    n80 = control-ref of="T1"() -> (w245:refnum<vi>)
    n81 = control-ref of="T2"() -> (w244:refnum<vi>)
    n82 = control-ref of="T3"() -> (w243:refnum<vi>)
    n83 = expression code="x*1000-100"(w271) -> (w273:dbl)
    n84 = Equal To 0?(x=w218) -> (x = 0?=w217:bool)
    n85 = Equal?(x=w220, y=w221) -> (x = y?=w219:bool)
    n86 = Build Array(w242) -> (w240:refnum<vi>[])
    n87 = Format Into String(format string="%d / %d", w220, w221) -> (resulting string=→"Run index":string)  [unwired: 2 in, 1 out]
    n88 = Build Array(w245, w244, w243) -> (w241:refnum<vi>[])
    n89 = Array Size(array=w267) -> (size(s)=w266:i32)
    n90 = To Unsigned Long Integer(number=w273) -> (unsigned 32bit integer=w274:u32)
    n91 = Initialize Array(10 ("element"), w266) -> (w222:i32[])
    n92 = call "Initialization_T_B_ver1.1.vi"("output cluster"=w268, "Measure with H/T sweep?"=w190, "First run?"=w217, "Last run?"=w219, "B Field Display Tex Array"=w240, "Temp. Display Ref Array"=w241) -> ("error out"=w281:errorcluster, "output cluster 2"=w282:T13, "Title Array"=w283:string[], "Comments String"=w215:string)  [unwired: 1 in]
    n93 = control-ref of="X"() -> (w263:refnum<vi>)
    n94 = control-ref of="Y 1"() -> (w262:refnum<vi>)
    n95 = control-ref of="Y 2"() -> (w261:refnum<vi>)
    n96 = control-ref of="Y 3"() -> (w260:refnum<vi>)
    n97 = control-ref of="Y 4"() -> (w259:refnum<vi>)
    n98 = control-ref of="Y 5"() -> (w258:refnum<vi>)
    n99 = control-ref of="Y 6"() -> (w257:refnum<vi>)
    n100 = Less Than 0?(x=w274) -> (x < 0?=w272:bool)
    n101 = local write "Description of this measurement"(w269) -> ()
    n102 = call "Initialization_Instru_ver1.0.vi"("error in (no error)"=w281, "output cluster"=w282, "Input Comments String"=w215, "T&B Title Array"=w283) -> ("error out"=w279:errorcluster, "output cluster 2"=w280:T13, "Output Comments String"=w214:string, "Title Array"=w223:string[])  [unwired: 1 in]
    "Title Name Array" <- w223
    n103 = Select(t=u32 0 ("unsigned 32bit integer"), s=w272, f=w274) -> (s? t:f=w270:u32)
    n104 = Build Array(w263, w262, w261, w260, w259, w258, w257) -> (w255:refnum<vi>[])
    n105 = control-ref of="XY Graph"() -> (w256:refnum<vi>)
    n106 = control-ref of="Scale"() -> (w254:refnum<vi>)
    n107 = call "DisplayBottomControl_DP_Ver5.0.vi"("Control Ring Array"=w255, "XYGraph Refnum"=w256, "Scale Arr Refnum"=w254, "Title Name Array"=w223) -> ("Y Ref. Output"=w253:refnum<vi>[], "dup Scale Arr Refnum"=w252:refnum<vi>, "XY WFGraph Ref."=w251:refnum<vi>)  [unwired: 2 in]
    n108 = call "InitialDelayCountdown_DP_Ver1.0.vi"("Temp. Display Ref Array"=w241, "output cluster"=w280, "error in"=w279, "B Field Display Tex Array"=w240) -> ("Stay duration pts"=w276:dbl[], "2D Array of DC Source or Lock-In Ctrl Run Cluster"=w278:cluster{"GPIB ADR":u16, "DC St. Pt.":dbl}[][], "output cluster 2"=w277:T13, "error out"=w238:errorcluster)  [unwired: 8 in]
    n109 = stacked-sequence {
      tunnel: [T14."Measurement" ("Tab Control")] -> w239
      tunnel: w238 -> [_]
      frame #0 {
      }
    }
    n110 = property on="Tab Control" class="TabCtl (strict)"("Value"=w239) -> ()  [unwired: 2 in, 2 out]
    n111 = property on="stop" class="Bool (strict)"("Value"=FALSE ("stop")) -> (error out=w248:errorcluster)  [unwired: 2 in, 1 out]
    n112 = property on="XY Graph" class="XYGraph (strict)"("Value"=cluster{"DataOut":dbl[], "DataOut":dbl[]}[] [] ("Value (Signaling)")) -> (error out=w247:errorcluster)  [unwired: 2 in, 1 out]
    n113 = property on="Data Table" class="Arr (strict)"("Value"=w264) -> (error out=w250:errorcluster)  [unwired: 2 in, 1 out]
    n114 = while {
      tunnel: w278 -> [w436]
      tunnel: w277 -> [w435]
      tunnel: w238 -> [w434]
      tunnel: w276 -> [w437]
      tunnel: w270 -> [w431]
      shift-right: [w410] -> w213
      shift-left: w264 -> [w412]
      tunnel: ["Description of this measurement"] -> w227
      tunnel: [w406] -> w207
      tunnel: w253 -> [w405]
      tunnel: w252 -> [w404]
      tunnel: w251 -> [w403]
      tunnel: w250 -> [_]
      tunnel: w248 -> [_]
      tunnel: w247 -> [_]
      tunnel: [w390] -> w225
      tunnel: [w394] -> w237
      tunnel: ["Data File Address"] -> w229
      tunnel: ["File Index:"] -> w228
      tunnel: [w389] -> w224
      tunnel: w222 -> [w387]
      i -> [w424]
      stop <- w432 stop-if-true
      w394 = FALSE
      # "Time_sec"
      n115 = call "InstruSweepControl_DP_ver1.0.vi"("Run Index"=w424, "error in"=w434, "output cluster"=w435, "2D Array of DC Source or Lock-In Ctrl Run Cluster"=w436, "Stay duration pts"=w437) -> ("error out"=w427:errorcluster, "output cluster 2"=w428:T13, "Run Stop?"=w429:bool, "Const I output"=w388:dbl[])  [unwired: 1 in]
      n116 = call "DisplayBottomColorVer_DP_2.0.vi"("WFGraph Ref."=w403, "Scale Arr Refnum"=w404, "Y Ref. Output"=w405) -> ()  [unwired: 3 in]
      n117 = Equal To 0?(x=w424) -> (x = 0?=w425:bool)
      n118 = case shown="True" w425 {
        tunnel: w424 -> [_ w447]
        tunnel: [w442 w447] -> w423
        tunnel: w421 -> [w441 w445]
        tunnel: [w441 w445] -> w420
        frame False {
          n119 = local read "StartTime(ms)"() -> (w443:u32)
          n120 = Tick Count (ms)() -> (millisecond timer value=w444:u32)
          n121 = Subtract(x=w444, y=w443) -> (x-y=w442:u32)
        }
        frame True {
          n122 = Tick Count (ms)() -> (millisecond timer value=→"StartTime(ms)":u32)
        }
      }
      n123 = Select(t=w424, s=w425, f=w431) -> (s? t:f=w430:u32)
      n124 = Or(x="stop", y=w429) -> (x .or. y?=w432:bool)
      n125 = flat-sequence {
        tunnel: w430 -> [w455]
        tunnel: w428 -> [w453]
        tunnel: w427 -> [w452]
        tunnel: [TRUE] -> w426
        tunnel: [w451] -> w419
        tunnel: [w450] -> w421
        frame #0 {
          n126 = call "FridgeStatusRead_ver1.0.vi"("error in"=w452, "output cluster"=w453) -> ("error out"=w450:errorcluster, "output cluster 2"=w451:T13, "Set B (T)"=→"Set B:":string, "Set T (K)"=→"Set T:":string)  [unwired: 2 in, 4 out]
          n127 = Wait (ms)(milliseconds to wait=w455) -> ()  [unwired: 1 out]
        }
      }
      n128 = To Double Precision Float(number=w423) -> (double precision float=w422:dbl)
      n129 = expression code="x/1000"(w422) -> (w414:dbl)
      n130 = call "InstruDataRead_DP_ver2.1.vi"("error in"=w420, "memory of # of pts in buffer"=w387, "Const I output"=w388, "output cluster"=w419) -> ("error out"=w391:errorcluster, "Data"=w413:dbl[], "output cluster 2"=w389:T13, "B (T)"=→"B":string, "T2 (K)"=→"T2":string, "T3 (K)"=→"T3":string, "T1 (K)"=→"T1":string)  [unwired: 1 out]
      n131 = while {
        tunnel: w391 -> [w440]
        tunnel: [w440] -> w390
        stop <- "Pause" continue-if-true
        n132 = Wait Until Next ms Multiple(millisecond multiple=u32 250) -> ()  [unwired: 1 out]
      }
      n133 = Build Array (concatenate)(w414, w413) -> (w411:dbl[])
      n134 = Build Array (concatenate)(w412, w411) -> (w410:dbl[][])
      "Data Table" <- w410
      n135 = control-ref of="Y 1"() -> (w397:refnum<vi>)
      n136 = control-ref of="Y 2"() -> (w398:refnum<vi>)
      n137 = control-ref of="Y 3"() -> (w399:refnum<vi>)
      n138 = control-ref of="Y 4"() -> (w400:refnum<vi>)
      n139 = control-ref of="Y 5"() -> (w401:refnum<vi>)
      n140 = control-ref of="Y 6"() -> (w402:refnum<vi>)
      n141 = Build Array(w397, w398, w399, w400, w401, w402) -> (w396:refnum<vi>[])
      n142 = local read "Title Name Array"() -> (w406:string[])
      n143 = call "MultiPlotting_6Plot_DPVer1.0.vi"("2D-DataIn"=w410, "DataDisplay Ref Array"=w396, "DisplayControl"="DisplayControl") -> ("DataDisplay"=→"DataDisplay":T11, "XY Graph"=→"XY Graph":cluster{"DataOut":dbl[], "DataOut":dbl[]}[])  [unwired: 3 in]
      n144 = local write "TakingData"(w394) -> ()
      "TakingData" <- w426
    }
    n145 = Strip Path(path=w229) -> (stripped path=w234:path, name=w233:string)
    n146 = local write "stop"(w237) -> ()
    n147 = local write "TakingData"(w237) -> ()
    n148 = call "CloseInstru.vi"("error in"=w225, "output cluster"=w224) -> ("error out"=w210:errorcluster, "output cluster 2"=w212:T13)
    n149 = Add(x=w228, y=w218) -> (x+y=w230:i32)
    n150 = Match Pattern(string=w233, regular expression=".itx") -> (before substring=w231:string)  [unwired: 1 in, 3 out]
    n151 = flat-sequence {
      tunnel: w197 -> [w290]
      tunnel: w196 -> [w286]
      tunnel: [w286] -> w195
      tunnel: w195 -> [w301]
      frame #0 {
        n152 = control-ref of="Scale"() -> (w291:refnum<vi>)
        n153 = control-ref of="X - axis"() -> (w300:refnum<vi>)
        n154 = control-ref of="Y 1"() -> (w299:refnum<vi>)
        n155 = control-ref of="Y 2"() -> (w298:refnum<vi>)
        n156 = control-ref of="Y 3"() -> (w297:refnum<vi>)
        n157 = control-ref of="Y 4"() -> (w296:refnum<vi>)
        n158 = control-ref of="Y 5"() -> (w295:refnum<vi>)
        n159 = control-ref of="Y 6"() -> (w294:refnum<vi>)
        n160 = Build Array(w300, w299, w298, w297, w296, w295, w294) -> (w292:refnum<vi>[])
        n161 = control-ref of="XY Graph 2"() -> (w293:refnum<vi>)
        n162 = call "DisplayBottomControl_DP_Ver5.0.vi"("Control Ring Array"=w292, "XYGraph Refnum"=w293, "Scale Arr Refnum"=w291, "Title Name Array"=w290) -> ("Y Ref. Output"=w289:refnum<vi>[], "dup Scale Arr Refnum"=w288:refnum<vi>, "XY WFGraph Ref."=w287:refnum<vi>)  [unwired: 2 in]
        n163 = call "DisplayBottomColorVer_DP_2.0.vi"("WFGraph Ref."=w287, "Scale Arr Refnum"=w288, "Y Ref. Output"=w289) -> ()  [unwired: 3 in]
      }
      frame #1 {
        n164 = call "MultiPlotting_6PlotForADC.vi"("2D-DataIn"=w301, "DisplayControl"="AnalysisDisplayControl") -> ("XY Graph"=→"XY Graph 2":cluster{"DataOut":dbl[], "DataOut":dbl[]}[])  [unwired: 4 in, 1 out]
      }
    }
    n165 = call "DataAveAnalysis.vi"("CernoxI measured with a lock-in?"="CernoxI measured with a lock-in?", "Title Name Array In"=w207, "Cernox_I"="Cernox_I", "2D Data Array In"=w213, "output cluster"=w212, "# of Discarded pts"="Discarded pts", "error in"=w210, "Cernox T Fitting Control"="Cernox T Fitting Control") -> ("Title Name Array Out"=w197:string[], "2D Data ArrayOut"=w208:dbl[][], "2D Data  Analysis"=w196:dbl[][], "Title Name Before Std"=w193:string[], "error out"=w211:errorcluster)  [unwired: 2 in, 1 out]
    n166 = Format Into String(format string="%03d.itx", initial string=w231, w230) -> (resulting string=w235:string)  [unwired: 1 in, 1 out]
    n167 = Build Path(base path=w234, name or relative path=w235) -> (appended path=w200:path)
    n168 = Strip Path(path=w200) -> (stripped path=w203:path, name=w201:string)
    n169 = Match Pattern(string=w201, regular expression=".itx") -> (before substring=w204:string)  [unwired: 1 in, 3 out]
    n170 = Concatenate Strings(w204, "_Sum.itx" ("regular expression")) -> (w206:string)
    n171 = Build Path(base path=w203, name or relative path=w206) -> (appended path=w199:path)
    n172 = case shown="0, Default" "File type" {
      tunnel: w200 -> [w310 w330 w351]
      tunnel: w193 -> [w309 w329 w350]
      tunnel: w227 -> [w314 w328 w349]
      tunnel: [w307 w323 w344] -> w226
      tunnel: w211 -> [w313 w327 w348]
      tunnel: w214 -> [w312 _ w347]
      tunnel: w208 -> [w311 w326 w343]
      tunnel: w197 -> [_ w321 w341]
      tunnel: w196 -> [w306 w322 w340]
      tunnel: w199 -> [w305 w325 w342]
      tunnel: "Analysis" -> [w304 w320 w338]
      frame 0, Default {
        # "txt"
        n173 = call "WriteTxtDataFile_DP_ver1.0.vi"("2D Data Array In"=w311, "Title Name Array"=w309, "error in"=w313, "Run Info. Comment"=w314, "Initial String"=w312, "file path"=w310) -> ("error out"=w308:errorcluster)  [unwired: 1 in]
        n174 = case shown="True" w304 {
          tunnel: w308 -> [w315 w319]
          tunnel: [w315 w318] -> w307
          tunnel: w306 -> [_ w317]
          tunnel: w305 -> [_ w316]
          frame False {
          }
          frame True {
            n175 = call "WriteTxtDataAnaFile_DP_ver1.0.vi"("2D Data Array In"=w317, "error in"=w319, "file path"=w316) -> ("error out"=w318:errorcluster)  [unwired: 4 in]
          }
        }
      }
      frame 1 {
        # "Igor"
        n176 = call "WriteIgorDataFile_DP_ver1.0.vi"("2D Data Array In"=w326, "Title Name Array"=w329, "error in"=w327, "Run Info. Comment"=w328, "file path"=w330) -> ("error out"=w324:errorcluster)  [unwired: 2 in]
        n177 = case shown="True" w320 {
          tunnel: w325 -> [_ w337]
          tunnel: w324 -> [w331 w336]
          tunnel: [w331 w335] -> w323
          tunnel: w322 -> [_ w334]
          tunnel: w321 -> [_ w333]
          frame False {
          }
          frame True {
            n178 = call "WriteIgorDataFile_DP_ver1.0.vi"("2D Data Array In"=w334, "Title Name Array"=w333, "error in"=w336, "Run Info. Comment"="Data Analysis File", "file path"=w337) -> ("error out"=w335:errorcluster)  [unwired: 2 in]
          }
        }
      }
      frame 2 {
        # "Both"
        n179 = stacked-sequence {
          tunnel: w351 -> [w362 w379]
          tunnel: w350 -> [w361 w380]
          tunnel: w349 -> [w360 w377]
          tunnel: [w354 _] -> w345
          tunnel: w348 -> [w359 w376]
          tunnel: w347 -> [_ w378]
          tunnel: w343 -> [w358 w375]
          tunnel: w342 -> [w356 w374]
          tunnel: w341 -> [w355 _]
          tunnel: w340 -> [w357 w371]
          tunnel: [_ w372] -> w339
          tunnel: w338 -> [w352 w370]
          frame #0 {
            n180 = call "WriteIgorDataFile_DP_ver1.0.vi"("2D Data Array In"=w358, "Title Name Array"=w361, "error in"=w359, "Run Info. Comment"=w360, "file path"=w362) -> ("error out"=w353:errorcluster)  [unwired: 2 in]
            n181 = case shown="True" w352 {
              tunnel: w357 -> [_ w368]
              tunnel: w356 -> [_ w367]
              tunnel: w355 -> [_ w366]
              tunnel: [w363 w365] -> w354
              tunnel: w353 -> [w363 w364]
              frame False {
              }
              frame True {
                n182 = call "WriteIgorDataFile_DP_ver1.0.vi"("2D Data Array In"=w368, "Title Name Array"=w366, "error in"=w364, "Run Info. Comment"="Data Analysis File", "file path"=w367) -> ("error out"=w365:errorcluster)  [unwired: 2 in]
              }
            }
          }
          frame #1 {
            n183 = call "WriteTxtDataFile_DP_ver1.0.vi"("2D Data Array In"=w375, "Title Name Array"=w380, "error in"=w376, "Run Info. Comment"=w377, "Initial String"=w378, "file path"=w379) -> ("error out"=w373:errorcluster)  [unwired: 1 in]
            n184 = case shown="True" w370 {
              tunnel: w374 -> [_ w385]
              tunnel: w373 -> [w381 w384]
              tunnel: [w381 w383] -> w372
              tunnel: w371 -> [_ w382]
              frame False {
              }
              frame True {
                n185 = call "WriteTxtDataAnaFile_DP_ver1.0.vi"("2D Data Array In"=w382, "error in"=w384, "file path"=w385) -> ("error out"=w383:errorcluster)  [unwired: 4 in]
              }
            }
          }
        }
        n186 = Build Array(w345, w339) -> (w346:errorcluster[])
        n187 = Merge Errors(w346) -> (w344:errorcluster)
      }
    }
    n188 = call <vilib>:"Simple Error Handler.vi"("error in (no error)"=w226) -> ()  [unwired: 4 in, 5 out]
  }
